vi "Day 14-Initialize Pair Count.vi"(11 "Initial Letters":u8[](array[numeric])) -> (3 "Map":map{u8[], u64}(c390))   [LabVIEW 2021]
uses:
  <vilib>/Utility/miscctls.llb/LVMapReplaceAction.ctl
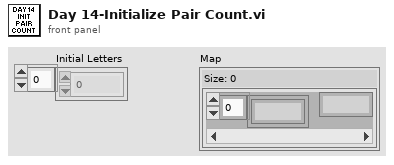
[diagram p1: front panel]
types:
  T1 = typedef "LVMapReplaceAction.ctl" = enum32{"Modify Entry only if found", "Add or Modify Entry", "Delete Entry"}
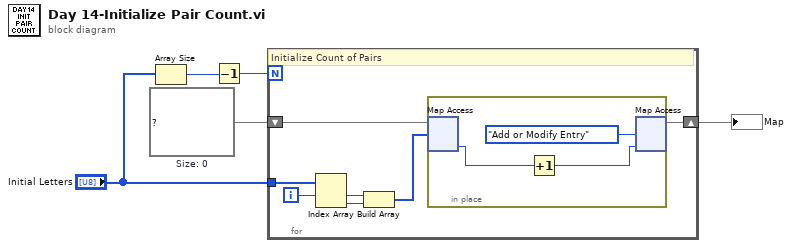
[diagram p0: block diagram]
diagram:
  w4 = map{u8[], u64} {}  # Size: 0
  n1 = Array Size(array="Initial Letters") -> (size(s)=w1:i32)
  n2 = Decrement(x=w1) -> (x-1=w2:i32)
  n3 = for {
    N: w2 -> [_]
    shift-right: [w10] -> w3
    shift-left: w4 -> [w9]
    tunnel: "Initial Letters" -> [w12]
    i -> [w11]
    # "Initialize Count of Pairs"
    n4 = Index Array(array=w12, index #1=w11) -> (element #1=w8:u8, element #2=w7:u8)  [unwired: 1 in]
    n5 = Build Array(w8, w7) -> (w6:u8[])
    n6 = in-place {
      n7 = in-place-map #1(w9, w6) -> (w14:u64)  [unwired: 1 in, 1 out]
      n8 = Increment(x=w14) -> (x+1=w13:u64)
      n9 = in-place-map #1(w13, LVMapReplaceAction."Add or Modify Entry" ("action")) -> (w10:map{u8[], u64})  [unwired: 2 out]
    }
  }
  "Map" <- w3
